vi "WPI_AnalogOutputRefNum Registry Get.vi"(8 "error in (no error)":errorcluster, 10 "refnum name":string="My AO RefNum") -> (0 "error out":errorcluster, 3 "AODeviceRef":T1={"DevStatus"={"status"=FALSE, "code"=0, "source"=""}, "AO Channel"=enum."Invalid"})   [LabVIEW 2017]
doc: "Gets the reference you specify. You first must set the reference with the RefNum Registry Set VI."
uses:
  <vilib>/Rock Robotics/WPI/AnalogOutput/WPI_AOChannelDevRef.ctl
  <vilib>/Rock Robotics/WPI/AnalogOutput/WPI_AnalogOutputChannel.ctl
  <vilib>/Rock Robotics/WPI/Utilities/Refnum Registry Operation.ctl
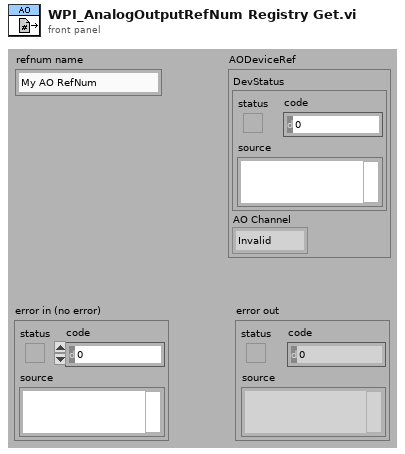
[diagram p1: front panel]
types:
  T1 = typedef "WPI_AOChannelDevRef.ctl" = cluster{"DevStatus":errorcluster, "AO Channel":T2}
  T2 = typedef "WPI_AnalogOutputChannel.ctl" = enum8{"AO MXP 0", "AO MXP 1", "Invalid"}
  T3 = typedef "Refnum Registry Operation.ctl" = enum16{"set", "get", "delete", "get all names", "read name"}
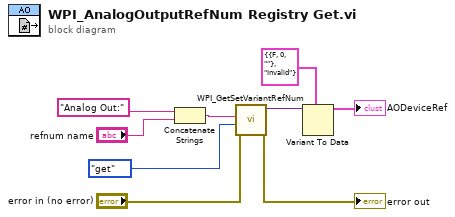
[diagram p0: block diagram]
diagram:
  n1 = Concatenate Strings("Analog Out:", "refnum name") -> (w4:string)
  n2 = call <vilib>:"WPI_GetSetVariantRefNum.vi"("error in (no error)"="error in (no error)", "Operation"=Refnum_Registry_Operation."get" ("menu"), "refnum name"=w4) -> ("error out"=→"error out":errorcluster, "DevRef"=w9:variant)  [unwired: 6 in, 1 out]
  n3 = Variant To Data(type=T1 {"DevStatus"={"status"=FALSE, "code"=0, "source"=""}, "AO Channel"=enum."Invalid"} ("AODeviceRef"), Variant=w9) -> (data=→"AODeviceRef":T1)  [unwired: 1 in, 1 out]
